vi "Array to String.vi"(10 "Input Array":dbl[](array[numeric])) -> (2 "CSV Result":string)   [LabVIEW 2013, in "BaseProducer.lvclass"]
doc: "This sub-VI converts a numeric array to a floating-point colon-delimited string with 12 significant digits of precision."
uses:
  BaseProducer.lvclass
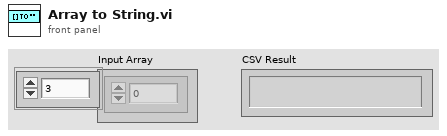
[diagram p1: front panel]
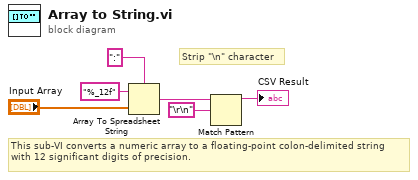
[diagram p0: block diagram]
diagram:
  # "Strip \"\\n\" character"
  # "This sub-VI converts a numeric array to a floating-point colon-delimited string with 12 significant digits of precision."
  n1 = Array To Spreadsheet String(delimiter (Tab)=":", array="Input Array", 3:"%_12f" ("format string")) -> (spreadsheet string=w3:string)
  n2 = Match Pattern(string=w3, regular expression="\r\n") -> (before substring=→"CSV Result":string)  [unwired: 1 in, 3 out]
